vi "Get Osc Support Sample Rates.vi"(8 "error in (no error)":errorcluster, 10 "maxnum":i32, 11 "sample":u32[](array[numeric])=[0, 0, 0, 0, 0, 0, 0, 0, 0, 0, 0, 0, 0, 0, 0, 0, 0, 0, 0, 0, 0, 0, 0, 0, 0, 0, 0, 0, 0, 0, 0, 0, 0, 0]) -> (0 "error out":errorcluster, 2 "function return":i32, 3 "sample out":u32[](array[numeric]))   [LabVIEW 2021, in "vmmso.lvlib"]
doc: "DLL_API int WINAPI GetOscSupportSampleRates(unsigned int* sample, int maxnum);"
uses:
  vmmso.lvlib
  vmmso.dll
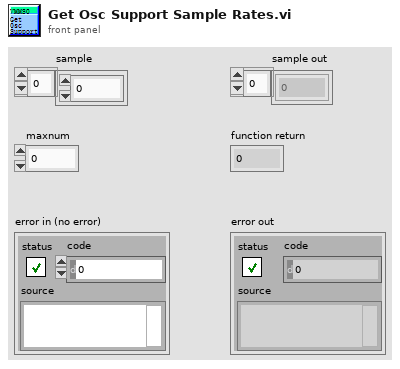
[diagram p1: front panel]
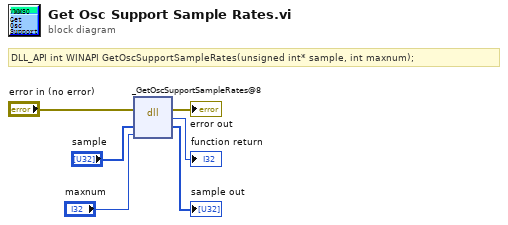
[diagram p0: block diagram]
diagram:
  # "DLL_API int WINAPI GetOscSupportSampleRates(unsigned int* sample, int maxnum);"
  n1 = dll-call lib="O:/MSO/library/demo-Labview/vmmso/vmmso.*" fn="_GetOscSupportSampleRates@8"(error in="error in (no error)", "sample"="sample", "maxnum"="maxnum") -> (error out=→"error out":errorcluster, →"function return":i32, "sample"=→"sample out":u32[])  [unwired: 3 in, 1 out]
